vi "Set Target Position - Absolute.vi"(4 "error in (no error)":errorcluster, 5 "Target Position":sgl, 6 "Axis In":i16, 7 "Controller Reference":refnum<k7>) -> (0 "error out":errorcluster, 2 "Axis Out":i16, 3 "Controller Reference out":refnum<k7>)   [LabVIEW 2015]
doc: "Sets the desired target position of the selected axis. Desired Position is an absolute position number NOT relative. Movement does not start until triggered by the DoGo command from a Start Movement type VI."
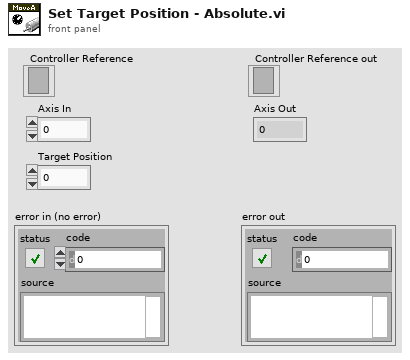
[diagram p1: front panel]
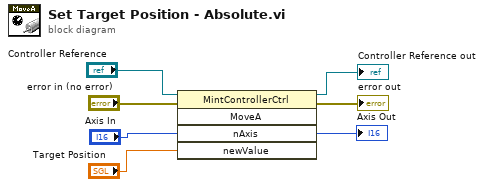
[diagram p0: block diagram]
diagram:
  n1 = invoke class="MintControllerCtrl" method="MoveA"(reference="Controller Reference", error in="error in (no error)", "nAxis"="Axis In", "newValue"="Target Position") -> (reference out=→"Controller Reference out":refnum<k7>, error out=→"error out":errorcluster, "nAxis"=→"Axis Out":i16)  [unwired: 1 in, 2 out]
